vi "D^.vi"(2 "D":bool, 3 "R":bool, 4 "^":bool) -> (0 "~Q":bool, 1 "Q":bool)   [LabVIEW 2019, in "Triggers.lvlib"]
uses:
  Triggers.lvlib
  Logik/Logik.lvlib
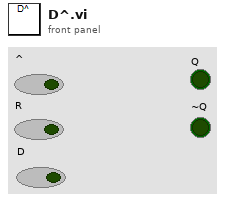
[diagram p1: front panel]
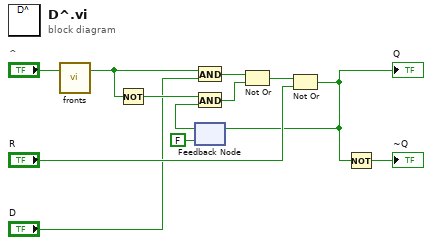
[diagram p0: block diagram]
diagram:
  n1 = call "fronts.vi"("in"="^") -> ("raise"=w1:bool)  [unwired: 1 in, 1 out]
  n2 = Not(x=w1) -> (.not. x?=w12:bool)
  n3 = And(x=w1, y="D") -> (x .and. y?=w10:bool)
  n4 = feedback #1(FALSE) -> (w11:bool)
  n5 = And(x=w12, y=w11) -> (x .and. y?=w9:bool)
  n6 = Not Or(1:w9, 2:w10) -> (0:w8:bool)
  n7 = Not Or(1:"R", 2:w8) -> (0:w6:bool)
  "Q" <- w6
  n8 = feedback-in #1(w6) -> ()
  n9 = Not(x=w6) -> (.not. x?=→"~Q":bool)
